vi "CH_LM App Resize Window.vi"(0 "menubar":refnum<k9>, 1 "item tag":string, 2 "i ref":refnum<vi>) -> ()   [LabVIEW 2012, in "CH_LM App.lvlib"]
doc: "This VI is used to resize the LabMax PC Frontpanel."
uses:
  CH_LM App.lvlib
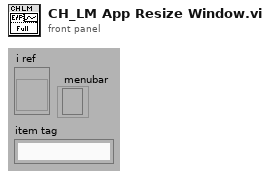
[diagram p1: front panel]
types:
  T1 = typedef "LVRectTypeDef.ctl" = cluster{"Left":i16, "Top":i16, "Right":i16, "Bottom":i16}
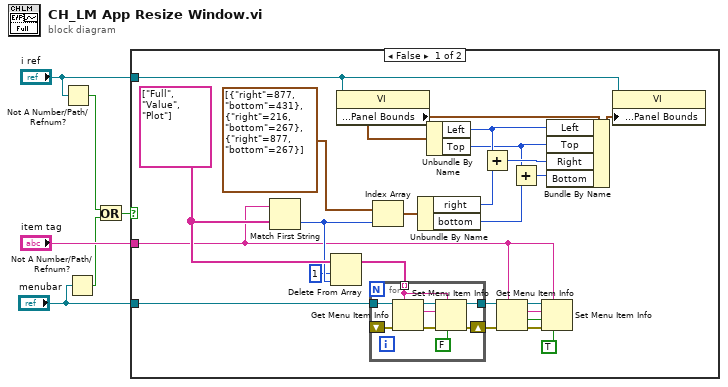
[diagram p0: block diagram]
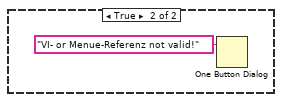
[diagram p2: hidden frame]
diagram:
  n1 = Not A Number/Path/Refnum?(number/path/refnum="i ref") -> (NaN/Path/Refnum?=w2:bool)
  n2 = Not A Number/Path/Refnum?(number/path/refnum="menubar") -> (NaN/Path/Refnum?=w1:bool)
  n3 = Or(x=w2, y=w1) -> (x .or. y?=w3:bool)
  n4 = case shown="False" w3 {
    tunnel: "i ref" -> [w10 _]
    tunnel: "item tag" -> [w9 _]
    tunnel: "menubar" -> [w8 _]
    frame False {
      w15 = string[] ["Full", "Value", "Plot"]
      n5 = Match First String(2:w15, 3:w9) -> (0:w14:i32)  [unwired: 1 out]
      n6 = Delete From Array(array=w15, length=1, index=w14) -> (array with subset deleted=w11:string[])  [unwired: 1 out]
      n7 = property class="VI"(reference=w10) -> ("Front Panel Window:Panel Bounds"=w29:T1)  [unwired: 1 in, 2 out]
      n8 = for {
        tunnel: w8 -> [w35]
        tunnel: [w34] -> w16
        shift-right: [w33] -> w12
        shift-left: _ -> [w31]
        tunnel: w11 -> [w32] mode=indexing
        n9 = Get Menu Item Info(7:w32, 8:w31, 11:w35) -> (0:w38:errorcluster, 2:w36:string, 3:w39:refnum<k9>)  [unwired: 4 out]
        n10 = Set Menu Item Info(6:FALSE ("checked"), 7:w32, 8:w38, 10:w36, 11:w39) -> (0:w33:errorcluster, 3:w34:refnum<k9>)  [unwired: 2 out]
      }
      n11 = Index Array(array=cluster{"right":i16, "bottom":i16}[] [{"right"=877, "bottom"=431}, {"right"=216, "bottom"=267}, {"right"=877, "bottom"=267}], index=w14) -> (element=w27:cluster{"right":i16, "bottom":i16})
      n12 = Unbundle By Name(w27) -> ("right"=w24:i16, "bottom"=w21:i16)
      n13 = Unbundle By Name(w29) -> ("Left"=w26:i16, "Top"=w22:i16)
      n14 = Add(x=w26, y=w24) -> (x+y=w25:i16)
      n15 = Get Menu Item Info(7:w9, 8:w12, 11:w16) -> (0:w18:errorcluster, 1:w7:bool, 2:w20:string, 3:w17:refnum<k9>)  [unwired: 3 out]
      n16 = Add(x=w22, y=w21) -> (x+y=w23:i16)
      n17 = Set Menu Item Info(6:TRUE ("checked"), 7:w9, 8:w18, 9:w7, 10:w20, 11:w17) -> ()  [unwired: 3 out]
      n18 = Bundle By Name(cluster=w29, "Left"=w26, "Top"=w22, "Right"=w25, "Bottom"=w23) -> (w28:T1)
      n19 = property class="VI"(reference=w10, "Front Panel Window:Panel Bounds"=w28) -> ()  [unwired: 1 in, 2 out]
    }
    frame True {
      n20 = One Button Dialog(message="VI- or Menue-Referenz not valid!") -> ()  [unwired: 2 out]
    }
  }
